vi "test VIT All Verifies With Labels.vi"(8 "error in":errorcluster, 11 "Testing Approval Tests in":refnum<class "VITester Extension Tests.lvclass">) -> (0 "error out":errorcluster, 3 "Testing Approval Tests in":refnum<class "VITester Extension Tests.lvclass">)   [LabVIEW 2026, in "VITester Extension Tests.lvclass"]
uses:
  VITester Extension Tests.lvclass
  Source/Approval Tests/Options/Options.lvclass/Options.ctl
  Source/Approval Tests/Naming Data/Naming Data.lvclass/Naming Data.ctl
  25835d91-223e-4457-8654-ed94975679ce.vi
  24d0000c-8485-4d5f-9e8a-c81d323cd4a2.vi
  1e735b7d-9815-499c-8608-d65425232398.vi
  1e735b7d-9815-499c-8608-d65425232398.vi/ef028380-787c-4fa5-86c8-b0b7860ce2dc.vi
  Source/Approval Tests/Replace if Empty.vi
  Source/Approval Tests/Update Test Name if Not Defined.vi
  Source/Approval Tests/Verify Core.vi
  1e735b7d-9815-499c-8608-d65425232398.vi/ef028380-787c-4fa5-86c8-b0b7860ce2dc.vi/93c5622b-9fb7-41e0-8c76-3fde37e94e34.vi
  Source/Approval Tests/Options/Read Scrubber.vi
  Source/Approval Tests/Naming Data/Read Test VI Name.vi
  Source/Approval Tests/Naming Data/Write Test VI Name.vi
  Source/Approval Tests/Options/Read Namer.vi
  Source/Approval Tests/Options/Read Naming Data.vi
  Source/Approval Tests/Options/Read Reporter.vi
  Source/Approval Tests/Options/Read Text Comparator.vi
  1e735b7d-9815-499c-8608-d65425232398.vi/ef028380-787c-4fa5-86c8-b0b7860ce2dc.vi/93c5622b-9fb7-41e0-8c76-3fde37e94e34.vi/04cb982b-2eda-40d0-8d7e-90f8e0b569b2.vi
  Source/Approval Tests/Options/Add Label to Namer.vi
  Source/Approval Tests/conv EOL.vi
  <vilib>/Utility/libraryn.llb/Check if File or Folder Exists.vi
  Source/Approval Tests/Reporter/Report.vi
  Caraya.Tests/Caraya Extension Tests/Utility Greet.vi
  Source/Approval Tests/Options/Options.lvclass
  Source/Approval Tests/Scrubber/Scrubber.lvclass
  Source/Approval Tests/Namer/Namer.lvclass
  Source/Approval Tests/Naming Data/Naming Data.lvclass
  Source/Approval Tests/Reporter/Reporter.lvclass
  Source/Approval Tests/Text Comparator/Text Comparator.lvclass
  VITester Extension Tests.lvclass/VITester Extension Tests.ctl
  Caraya.Tests/Caraya Extension Tests/Caraya Extension Tests.lvclass
  Source/Extensions/VITester.Extension/VITester.Extension.lvlib
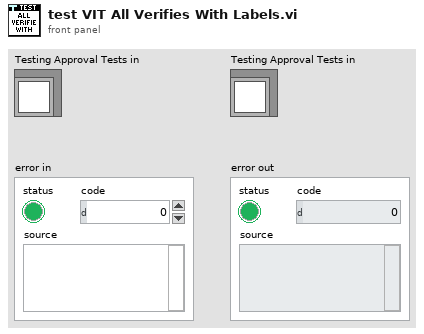
[diagram p1: front panel]
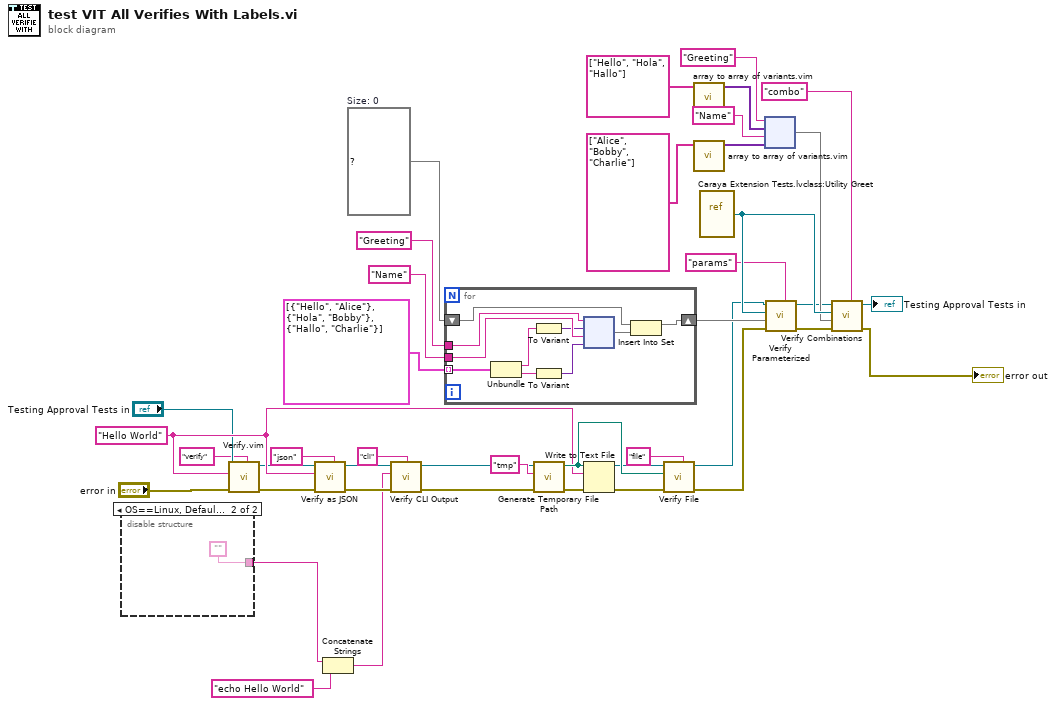
[diagram p0: block diagram]
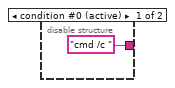
[diagram p2: hidden frame]
diagram:
  w31 = set{map{string, variant}} {}  # Size: 0
  w17 = "Hello World"
  n1 = disable-structure shown="OS==Linux, Default" {
    disable-tunnel: ["cmd /c " ""] -> w2
    frame condition #0 (active) {
    }
    frame condition #1 {
    }
  }
  n2 = call "Verify.vim"("Label"="verify", "error in"="error in", "Test Data"=w17, "TestCase in"="Testing Approval Tests in") -> ("error out"=w41:errorcluster, "TestCase out"=w15:refnum<class "VITester Extension Tests.lvclass">)  [unwired: 6 in]
  n3 = call "Verify as JSON.vi"("Label"="json", "error in"=w41, "Anything"=w17, "TestCase in"=w15) -> ("error out"=w40:errorcluster, "TestCase out"=w14:refnum<class "VITester Extension Tests.lvclass">)  [unwired: 6 in]
  n4 = Concatenate Strings(w2, "echo Hello World" ("string")) -> (w1:string)
  n5 = call "Verify CLI Output.vi"("Label"="cli", "error in"=w40, "command line"=w1, "TestCase in"=w14) -> ("error out"=w37:errorcluster, "TestCase out"=w13:refnum<class "VITester Extension Tests.lvclass">)  [unwired: 6 in]
  n6 = for {
    tunnel: "Greeting" -> [w53]
    tunnel: cluster{string, string}[] [{"Hello", "Alice"}, {"Hola", "Bobby"}, {"Hallo", "Charlie"}] -> [w51] mode=indexing
    tunnel: "Name" -> [w52]
    shift-right: [w45] -> w32
    shift-left: w31 -> [w44]
    n7 = Unbundle(w51) -> (w50:string, w49:string)
    n8 = To Variant(anything=w50) -> (Variant=w47:variant)
    n9 = To Variant(anything=w49) -> (Variant=w46:variant)
    n10 = node ("Build Map")(w53, w47, w52, w46) -> (w48:map{string, variant})
    n11 = Insert Into Set(10:w48, 11:w44) -> (3:w45:set{map{string, variant}})  [unwired: 1 out]
  }
  n12 = call <vilib>:"Generate Temporary File Path.vi"("error in (no error)"=w37, "Temporary File Extension (tmp)"="tmp") -> ("error out"=w36:errorcluster, "Unique Temporary File Path"=w18:path)  [unwired: 8 in]
  n13 = Write to Text File(file (use dialog)=w18, text=w17, error in=w36) -> (error out=w35:errorcluster)  [unwired: 1 in, 2 out]
  n14 = call "Verify File.vi"("Label"="file", "error in"=w35, "Path to Binary File to Verify"=w18, "TestCase in"=w13) -> ("error out"=w39:errorcluster, "TestCase out"=w12:refnum<class "VITester Extension Tests.lvclass">)  [unwired: 6 in]
  n15 = call "array to array of variants.vim"("Array in"=string[] ["Hello", "Hola", "Hallo"]) -> ("Array out"=w23:variant[])  [unwired: 10 in]
  n16 = call "array to array of variants.vim"("Array in"=string[] ["Alice", "Bobby", "Charlie"]) -> ("Array out"=w24:variant[])  [unwired: 10 in]
  n17 = vi-ref "Caraya Extension Tests.lvclass:Utility Greet.vi"() -> (w27:refnum<vi>)
  n18 = node ("Build Map")("Greeting" ("key"), w23, "Name" ("key"), w24) -> (w26:map{string, variant[]})
  n19 = call "Verify Parameterized.vi"("Label"="params", "error in"=w39, "Set of ctl label -> value var"=w32, "VI in"=w27, "TestCase in"=w12) -> ("error out"=w38:errorcluster, "TestCase out"=w11:refnum<class "VITester Extension Tests.lvclass">)  [unwired: 5 in]
  n20 = call "Verify Combinations.vi"("Label"="combo", "error in"=w38, "ctl label -> value var[]"=w26, "VI Refnum"=w27, "TestCase in"=w11) -> ("error out"=→"error out":errorcluster, "TestCase out"=→"Testing Approval Tests in":refnum<class "VITester Extension Tests.lvclass">)  [unwired: 5 in]
